vi "Write Max Size.vi"(8 "error in (no error)":errorcluster, 10 "Max Size":cluster{"Width":i32, "Height":i32}, 11 "Dialog.lvclass in":refnum<class "Dialog.lvclass">) -> (0 "error out":errorcluster, 3 "Dialog.lvclass out":refnum<class "Dialog.lvclass">)   [LabVIEW 2012, in "Dialog.lvlib" / "Dialog.lvclass"]
uses:
  Dialog.lvclass
  Dialog.lvclass/Dialog.ctl
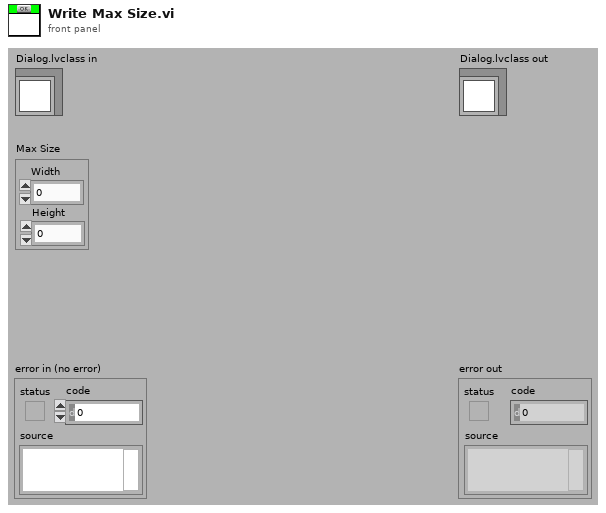
[diagram p1: front panel]
types:
  T1 = typedef "LVRectTypeDef.ctl" = cluster{"Left":i16, "Top":i16, "Right":i16, "Bottom":i16}
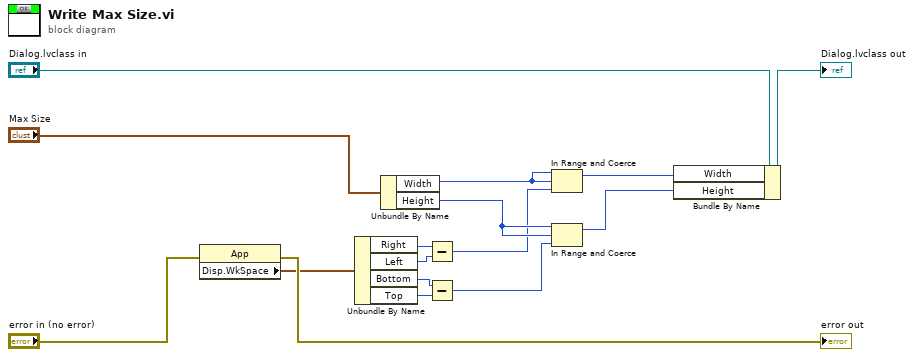
[diagram p0: block diagram]
diagram:
  n1 = property class="App"(error in="error in (no error)") -> (error out=→"error out":errorcluster, "Disp.WkSpace"=w1:T1)  [unwired: 1 in, 1 out]
  n2 = Unbundle By Name(w1) -> ("Right"=w11:i16, "Left"=w10:i16, "Bottom"=w8:i16, "Top"=w9:i16)
  n3 = Unbundle By Name("Max Size") -> ("Width"=w7:i32, "Height"=w5:i32)
  n4 = Subtract(x=w11, y=w10) -> (x-y=w3:i16)
  n5 = Subtract(x=w8, y=w9) -> (x-y=w2:i16)
  n6 = In Range and Coerce(upper limit=w7, x=w7, lower limit=w3) -> (coerced(x)=w6:i32)  [unwired: 1 out]
  n7 = In Range and Coerce(upper limit=w5, x=w5, lower limit=w2) -> (coerced(x)=w4:i32)  [unwired: 1 out]
  n8 = Bundle By Name(cluster="Dialog.lvclass in", "Width"=w6, "Height"=w4) -> (→"Dialog.lvclass out":refnum<class "Dialog.lvclass">)
